vi "FGV - Attocube Status.vi"(4 "error in":errorcluster, 6 "Function":enum16{"write", "read"}(ring), 7 "Status IN":T1) -> (0 "error out":errorcluster, 3 "Status OUT":T1)   [LabVIEW 2013]
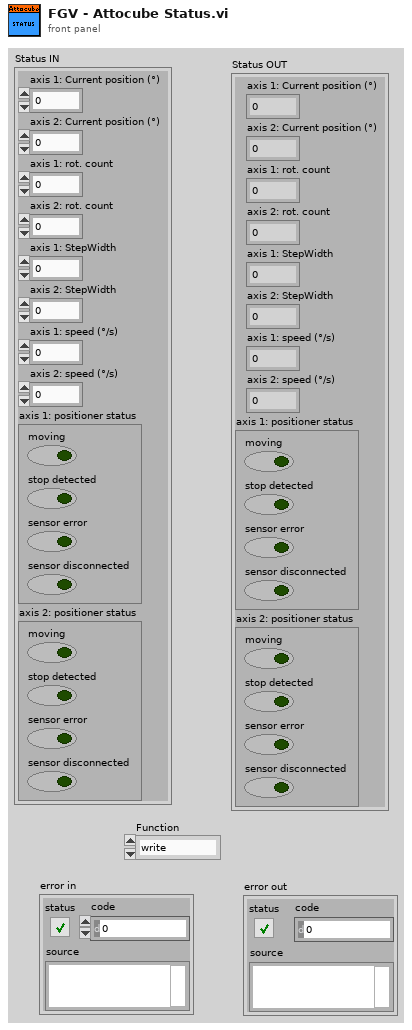
[diagram p1: front panel]
types:
  T1 = cluster{"axis 1: Current position (°)":dbl, "axis 2: Current position (°)":dbl, "axis 1: rot. count":dbl, "axis 2: rot. count":dbl, "axis 1: StepWidth":dbl, "axis 2: StepWidth":dbl, "axis 1: speed (°/s)":dbl, "axis 2: speed (°/s)":dbl, "axis 1: positioner status":cluster{"moving":bool, "stop detected":bool, "sensor error":bool, "sensor disconnected":bool}, "axis 2: positioner status":cluster{"moving":bool, "stop detected":bool, "sensor error":bool, "sensor disconnected":bool}}
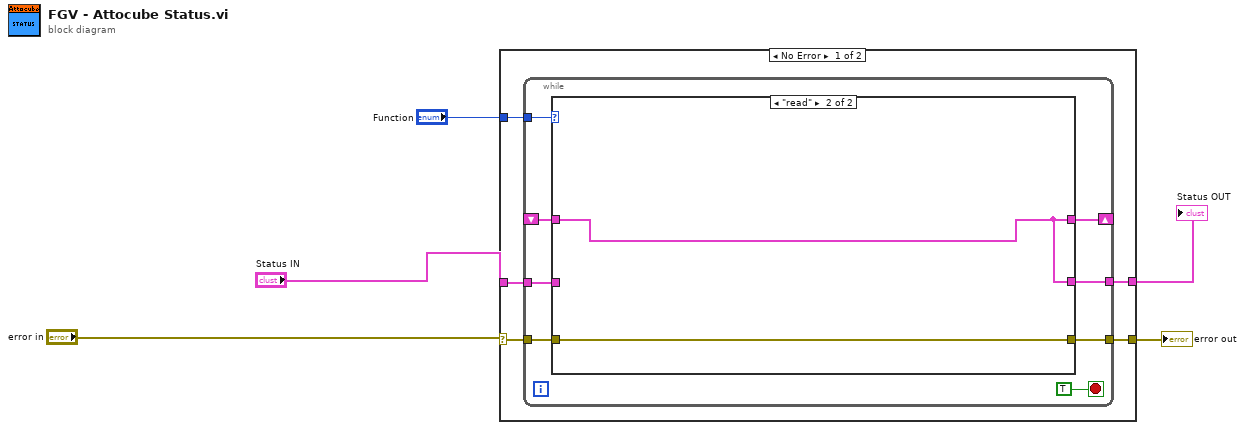
[diagram p0: block diagram]
diagram:
  n1 = case shown="No Error" "error in" {
    selector: "error in" -> [w10 w24]
    tunnel: [w9 w24] -> w5
    tunnel: [w8 w23] -> w2
    tunnel: "Function" -> [w7 _]
    tunnel: "Status IN" -> [w6 w23]
    frame No Error {
      n2 = while {
        shift-right: [w13] -> _
        shift-left: _ -> [w12]
        tunnel: w10 -> [w17]
        tunnel: [w16] -> w9
        tunnel: [w15] -> w8
        tunnel: w7 -> [w14]
        tunnel: w6 -> [w11]
        stop <- TRUE stop-if-true
        n3 = case shown="\"read\"" w14 {
          tunnel: w17 -> [w19 w21]
          tunnel: [w19 w21] -> w16
          tunnel: [w20 w22] -> w15
          tunnel: [w20 w22] -> w13
          tunnel: w12 -> [_ w22]
          tunnel: w11 -> [w20 _]
          frame "write", Default {
          }
          frame "read" {
          }
        }
      }
    }
    frame Error {
    }
  }
  "error out" <- w5
  "Status OUT" <- w2
